vi "DriverStationGetInstructions.vi"() -> ()   [LabVIEW 2019]
doc: "This VI receives instructions from the driver and manipulator controls, but only in certain robot modes. Specifically, these instructions are received while the robot is either \"running autonomously\" or in Super Test Mode. In all other robot modes, no instructions are received via the driver station. Instead they are output by the Autonomous Sequencer or completely disabled."
uses:
  refnums.vi
  dsinstructions.vi
  <vilib>/Rock Robotics/Network Tables/NT Read Boolean Array.vi
  dsdata.vi
  GRNF_Joystick.vi
  <vilib>/Rock Robotics/Network Tables/NT Read Boolean.vi
panel:
  in  "Buttons":bool[](array[boolean])=[FALSE, FALSE, FALSE, FALSE, FALSE, FALSE, FALSE, FALSE, FALSE, FALSE]
  in  "Right Trigger":dbl(slide) min=0.0 max=1.0 scale=0.0..1.0
  in  "Left Trigger":dbl(slide) min=0.0 max=1.0 step=0.1 scale=0.0..1.0
  in  "Right Joystick X":dbl(slide) scale=-1.0..1.0
  in  "Enable Joystick Control Override":bool
  in  "Joystick Left X":dbl(slide) scale=-1.0..1.0
  in  "Joystick Left Y":dbl(slide) scale=1.0..-1.0
  in  "Joystick Right Y":dbl(slide) scale=1.0..-1.0
  # "Left Thumbstick"
  # "Right Thumbstick"
  # "Driver A"
  # "Driver B"
  # "Driver X"
  # "Driver Y"
  # "Driver Left Bumper"
  # "Driver Right Bumper"
  # "Driver View"
  # "Driver Menu"
  # "Driver Left Joystick Button"
  # "Driver Right Joystick Button"
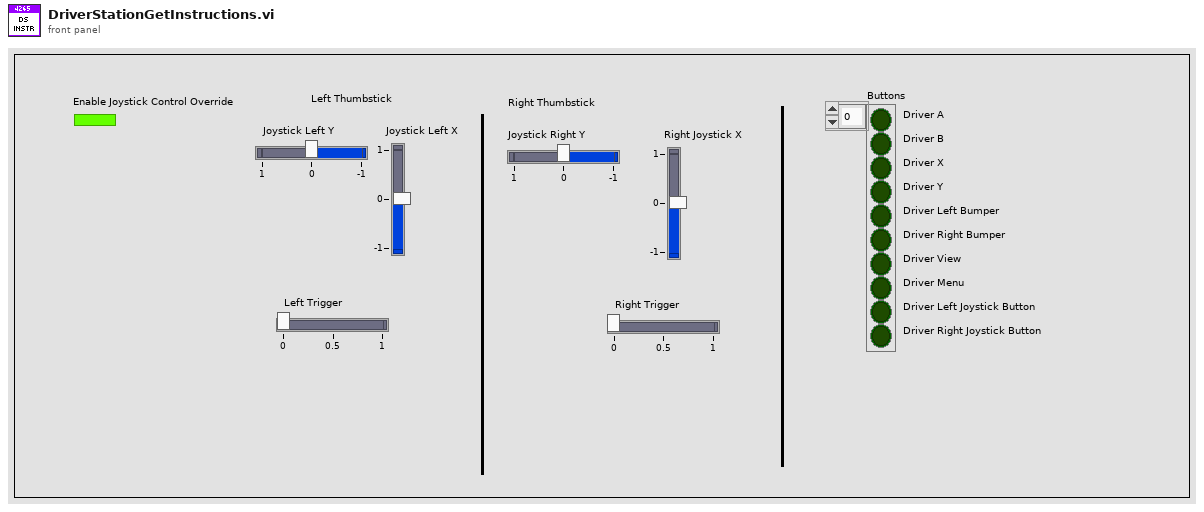
[diagram p1: front panel]
types:
  T1 = typedef "WPI_JoystickDevRef.ctl" = cluster{"Device":T2}
  T2 = typedef "WPI_JoystickDeviceEnum.ctl" = enum16{"USB 0", "USB 1", "USB 2", "USB 3", "USB 4", "USB 5"}
  T3 = enum16{"Center", "North", "NorthWest", "West", "SouthWest", "South", "SouthEast", "East", "NorthEast"}
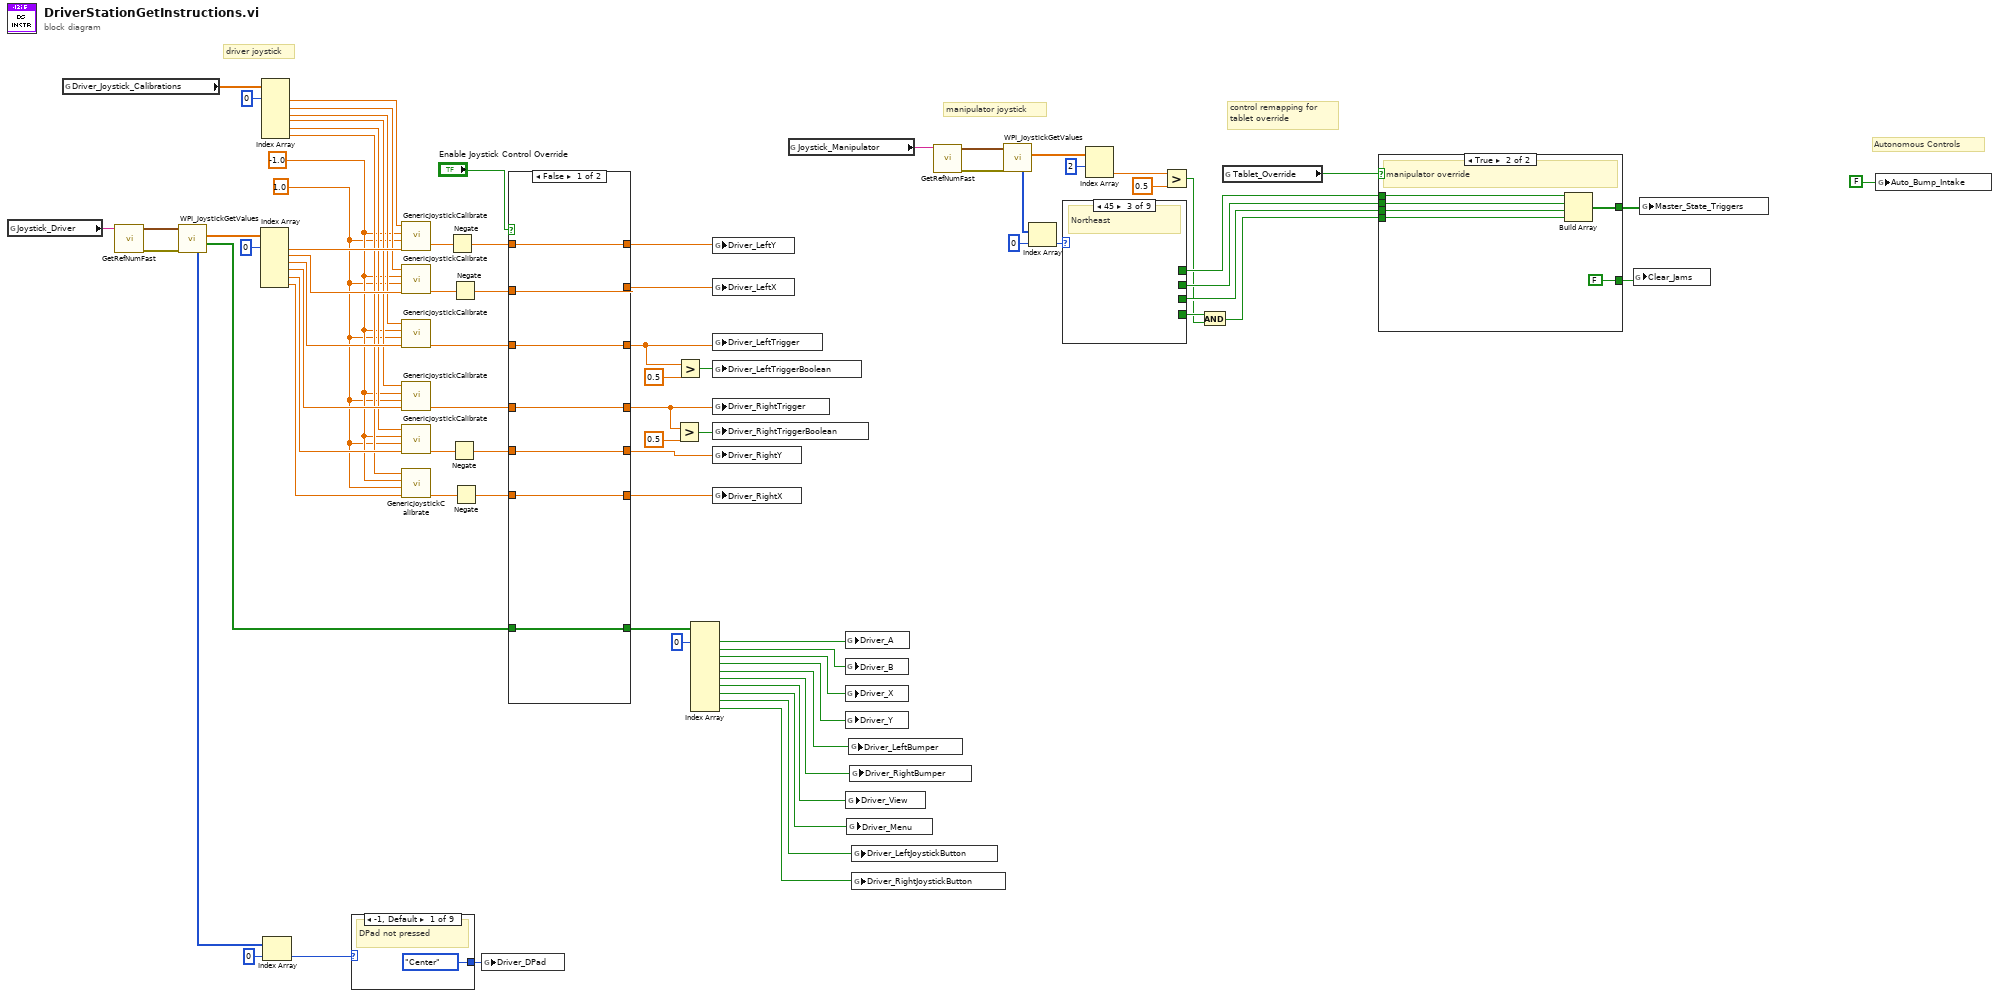
[diagram p0: block diagram]
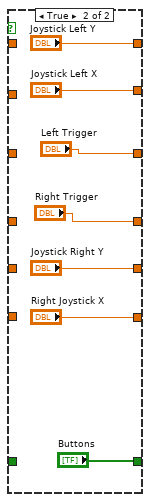
[diagram p2: hidden frame]
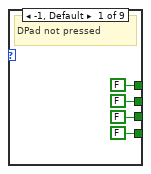
[diagram p3: hidden frame]
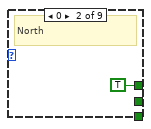
[diagram p4: hidden frame]
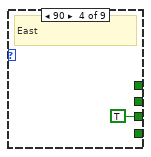
[diagram p5: hidden frame]
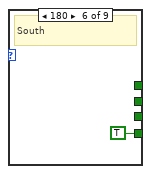
[diagram p7: hidden frame]
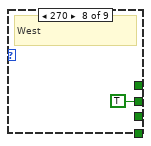
[diagram p9: hidden frame]
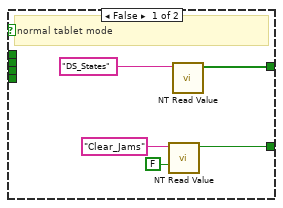
[diagram p11: hidden frame]
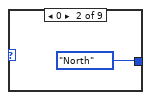
[diagram p12: hidden frame]
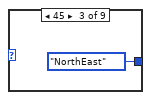
[diagram p13: hidden frame]
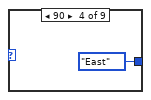
[diagram p14: hidden frame]
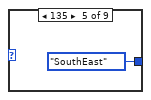
[diagram p15: hidden frame]
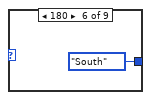
[diagram p16: hidden frame]
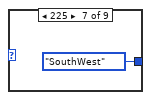
[diagram p17: hidden frame]
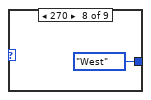
[diagram p18: hidden frame]
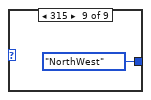
[diagram p19: hidden frame]
diagram:
  w20 = 1.0
  w21 = -1.0
  # "Autonomous Controls"
  # "control remapping for\ntablet override"
  # "manipulator joystick"
  # "driver joystick"
  n1 = global read "refnums.vi" "Joystick_Driver"() -> (w45:string)
  n2 = global read "dsdata.vi" "Driver_Joystick_Calibrations"() -> (w39:dbl[])
  n3 = call-poly "GetRefNumFast.vi"("RefNum Name"=w45) -> ("Error"=w46:errorcluster, "Device Reference"=w47:T1)  [unwired: 5 in]
  n4 = call <vilib>:"WPI_JoystickGetValues.vi"("error in (no error)"=w46, "JoystickDevRef"=w47) -> ("Buttons"=w2:bool[], "Axes"=w79:dbl[], "POVs"=w76:i16[])  [unwired: 5 in, 2 out]
  n5 = Index Array(array=w79, index #1=0 ("index")) -> (element #1=w33:dbl, element #2=w32:dbl, element #3=w28:dbl, element #4=w29:dbl, element #5=w30:dbl, element #6=w31:dbl)  [unwired: 5 in]
  n6 = Index Array(array=w39, index #1=0 ("index")) -> (element #1=w22:dbl, element #2=w23:dbl, element #3=w24:dbl, element #4=w25:dbl, element #5=w26:dbl, element #6=w27:dbl)  [unwired: 5 in]
  n7 = Index Array(array=w76, index=0) -> (element=w64:i16)
  n8 = case shown="-1, Default" w64 {
    tunnel: [T3."Center" T3."North" T3."NorthEast" T3."East" T3."SouthEast" T3."South" T3."SouthWest" T3."West" T3."NorthWest"] -> w63
    frame -1, Default {
      # "DPad not pressed"
    }
    frame 0 {
    }
    frame 45 {
    }
    frame 90 {
    }
    frame 135 {
    }
    frame 180 {
    }
    frame 225 {
    }
    frame 270 {
    }
    frame 315 {
    }
  }
  n9 = call "GenericJoystickCalibrate.vi"("Raw Joystick Value"=w33, "Maximum"=w20, "Minimum"=w21, "Deadband"=w22) -> ("Scaled Joystick Value"=w37:dbl)  [unwired: 3 in]
  n10 = call "GenericJoystickCalibrate.vi"("Raw Joystick Value"=w32, "Maximum"=w20, "Minimum"=w21, "Deadband"=w23) -> ("Scaled Joystick Value"=w36:dbl)  [unwired: 3 in]
  n11 = call "GenericJoystickCalibrate.vi"("Raw Joystick Value"=w28, "Maximum"=w20, "Minimum"=w21, "Deadband"=w24) -> ("Scaled Joystick Value"=w14:dbl)  [unwired: 3 in]
  n12 = call "GenericJoystickCalibrate.vi"("Raw Joystick Value"=w29, "Maximum"=w20, "Minimum"=w21, "Deadband"=w25) -> ("Scaled Joystick Value"=w8:dbl)  [unwired: 3 in]
  n13 = call "GenericJoystickCalibrate.vi"("Raw Joystick Value"=w30, "Maximum"=w20, "Minimum"=w21, "Deadband"=w26) -> ("Scaled Joystick Value"=w35:dbl)  [unwired: 3 in]
  n14 = call "GenericJoystickCalibrate.vi"("Raw Joystick Value"=w31, "Maximum"=w20, "Minimum"=w21, "Deadband"=w27) -> ("Scaled Joystick Value"=w34:dbl)  [unwired: 3 in]
  n15 = Negate(x=w37) -> (-x=w17:dbl)
  n16 = Negate(x=w35) -> (-x=w5:dbl)
  n17 = Negate(x=w36) -> (-x=w16:dbl)
  n18 = Negate(x=w34) -> (-x=w4:dbl)
  n19 = global write "dsinstructions.vi" "Driver_DPad"(w63) -> ()
  n20 = case shown="False" "Enable Joystick Control Override" {
    tunnel: w14 -> [w93 _]
    tunnel: [w95 "Joystick Left Y"] -> w18
    tunnel: w17 -> [w95 _]
    tunnel: [w94 "Joystick Left X"] -> w15
    tunnel: w16 -> [w94 _]
    tunnel: [w93 "Left Trigger"] -> w9
    tunnel: w8 -> [w92 _]
    tunnel: [w92 "Right Trigger"] -> w7
    tunnel: [w91 "Joystick Right Y"] -> w6
    tunnel: w5 -> [w91 _]
    tunnel: [w90 "Right Joystick X"] -> w3
    tunnel: w4 -> [w90 _]
    tunnel: w2 -> [w89 _]
    tunnel: [w89 "Buttons"] -> w1
    frame False {
    }
    frame True {
    }
  }
  n21 = Greater?(x=w7, y=0.5) -> (0:w11:bool)
  n22 = Greater?(x=w9, y=0.5) -> (0:w10:bool)
  n23 = Index Array(array=w1, index #1=0 ("index")) -> (element #1=w74:bool, element #2=w73:bool, element #3=w72:bool, element #4=w71:bool, element #5=w70:bool, element #6=w69:bool, element #7=w68:bool, element #8=w67:bool, element #9=w66:bool, element #10=w65:bool)  [unwired: 9 in]
  n24 = global write "dsinstructions.vi" "Driver_LeftY"(w18) -> ()
  n25 = global write "dsinstructions.vi" "Driver_LeftX"(w15) -> ()
  n26 = global write "dsinstructions.vi" "Driver_LeftTrigger"(w9) -> ()
  n27 = global write "dsinstructions.vi" "Driver_LeftTriggerBoolean"(w10) -> ()
  n28 = global write "dsinstructions.vi" "Driver_RightTrigger"(w7) -> ()
  n29 = global write "dsinstructions.vi" "Driver_RightTriggerBoolean"(w11) -> ()
  n30 = global write "dsinstructions.vi" "Driver_RightY"(w6) -> ()
  n31 = global write "dsinstructions.vi" "Driver_RightX"(w3) -> ()
  n32 = global read "refnums.vi" "Joystick_Manipulator"() -> (w42:string)
  n33 = global write "dsinstructions.vi" "Driver_A"(w74) -> ()
  n34 = global write "dsinstructions.vi" "Driver_B"(w73) -> ()
  n35 = global write "dsinstructions.vi" "Driver_X"(w72) -> ()
  n36 = global write "dsinstructions.vi" "Driver_Y"(w71) -> ()
  n37 = global write "dsinstructions.vi" "Driver_View"(w68) -> ()
  n38 = global write "dsinstructions.vi" "Driver_Menu"(w67) -> ()
  n39 = global write "dsinstructions.vi" "Driver_LeftBumper"(w70) -> ()
  n40 = global write "dsinstructions.vi" "Driver_RightBumper"(w69) -> ()
  n41 = global write "dsinstructions.vi" "Driver_LeftJoystickButton"(w66) -> ()
  n42 = global write "dsinstructions.vi" "Driver_RightJoystickButton"(w65) -> ()
  n43 = call-poly "GetRefNumFast.vi"("RefNum Name"=w42) -> ("Error"=w43:errorcluster, "Device Reference"=w44:T1)  [unwired: 5 in]
  n44 = call <vilib>:"WPI_JoystickGetValues.vi"("error in (no error)"=w43, "JoystickDevRef"=w44) -> ("Axes"=w62:dbl[], "POVs"=w55:i16[])  [unwired: 5 in, 3 out]
  n45 = Index Array(array=w55, index=0) -> (element=w56:i16)
  n46 = case shown="45" w56 {
    tunnel: [FALSE TRUE _ _ _ _ _ _ _] -> w54
    tunnel: [FALSE _ _ _ _ _ _ TRUE _] -> w53
    tunnel: [FALSE _ _ TRUE _ _ _ _ _] -> w52
    tunnel: [FALSE _ _ _ _ TRUE _ _ _] -> w51
    frame -1, Default {
      # "DPad not pressed"
    }
    frame 0 {
      # "North"
    }
    frame 45 {
      # "Northeast"
    }
    frame 90 {
      # "East"
    }
    frame 135 {
      # "Southeast"
    }
    frame 180 {
      # "South"
    }
    frame 225 {
      # "Southwest"
    }
    frame 270 {
      # "West"
    }
    frame 315 {
      # "Northwest"
    }
  }
  n47 = Index Array(array=w62, index #1=2 ("index")) -> (element #2=w60:dbl)  [unwired: 1 in, 1 out]
  n48 = Greater?(x=w60, y=0.5) -> (0:w49:bool)
  n49 = And(x=w51, y=w49) -> (x .and. y?=w50:bool)
  n50 = global read "dsdata.vi" "Tablet_Override"() -> (w48:bool)
  n51 = case shown="True" w48 {
    tunnel: [w114 w121] -> w58
    tunnel: w54 -> [_ w120]
    tunnel: w53 -> [_ w119]
    tunnel: w52 -> [_ w118]
    tunnel: w50 -> [_ w117]
    tunnel: [w111 FALSE ("Boolean")] -> w41
    frame False {
      # "normal tablet mode"
      n52 = call-poly <vilib>:"NT Read Value.vi"("Default Value"=FALSE, "Name"="Clear_Jams" ("refnum name")) -> ("Boolean"=w111:bool)  [unwired: 8 in, 1 out]
      n53 = call-poly <vilib>:"NT Read Value.vi"("Name"="DS_States" ("refnum name")) -> ("Boolean Array"=w114:bool[])  [unwired: 9 in, 1 out]
    }
    frame True {
      # "manipulator override"
      n54 = Build Array(w120, w119, w118, w117) -> (w121:bool[])
    }
  }
  n55 = global write "dsinstructions.vi" "Clear_Jams"(w41) -> ()
  n56 = global write "dsinstructions.vi" "Master_State_Triggers"(w58) -> ()
  n57 = global write "dsinstructions.vi" "Auto_Bump_Intake"(FALSE ("Auto_Bump_Intake")) -> ()
